vi "Close Subscription Policy.vi"(8 "error in (no error)":errorcluster, 11 "Subscription Policy Reference":T1) -> (0 "error out (Unsubscribe?)":errorcluster)   [LabVIEW 2015]
doc: "This method decides whether or not to send or otherwise handle the new data value. The policy is set and maintained by the subscriber. The Topic Actor knows no policy details, it just passes the new value in. If there is a failure inside this method, the Topic Actor must assume the listener is no longer valid (dead/unrecoverable) and should delete it from the Subscriber list.\n\n<License>\nCopyright © 2017 Composed Systems, LLC | All rights reserved\nwww.composed.io\n\nAuthor: Ethan Stern <ethan.stern@composed.io>\n\nThis software is provided \"AS IS\" WITHOUT WARRANTIES, either express or implied, AND IS FOR EDUCATIONAL PURPOSES ONLY.\n</License>"
uses:
  BasicSubscription.lvclass
  ISubscriptionPolicy Reference.ctl
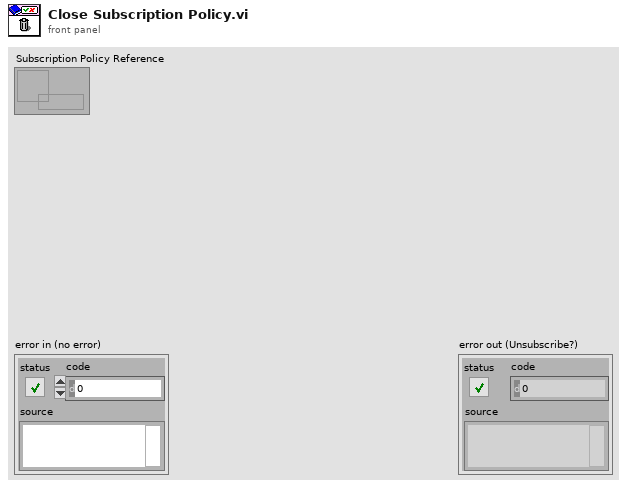
[diagram p1: front panel]
types:
  T1 = typedef "ISubscriptionPolicy Reference.ctl" = refnum<data-value>
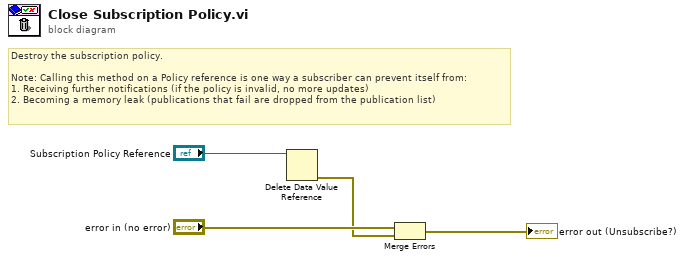
[diagram p0: block diagram]
diagram:
  # "Destroy the subscription policy.\n\nNote: Calling this method on a Policy reference is one way a subscriber can prevent itself from:\n1. Receiving further notifications (if the policy is invalid, no more updates)\n2. Becoming a memory leak (publications that fail are dropped from the publication list)"
  n1 = Delete Data Value Reference(data value reference="Subscription Policy Reference") -> (error out=w1:errorcluster)  [unwired: 1 in, 1 out]
  n2 = Merge Errors("error in (no error)", w1) -> (→"error out (Unsubscribe?)":errorcluster)
